vi "pp_loadStimParam.vi"(0 "error in (no error)":errorcluster) -> (5 "error out":errorcluster, 8 "Path":path, 14 "Total Trials":i32, 15 "Trial Randomization":enum32{"50% exactly", "Radio Selection 2"}(radio), 18 "Stims 1":dbl[][](array[numeric]), 19 "Stims 2":dbl[][](array[numeric]))   [LabVIEW 2013]
uses:
  <vilib>/Utility/xml.llb/Read From XML File(array).vi
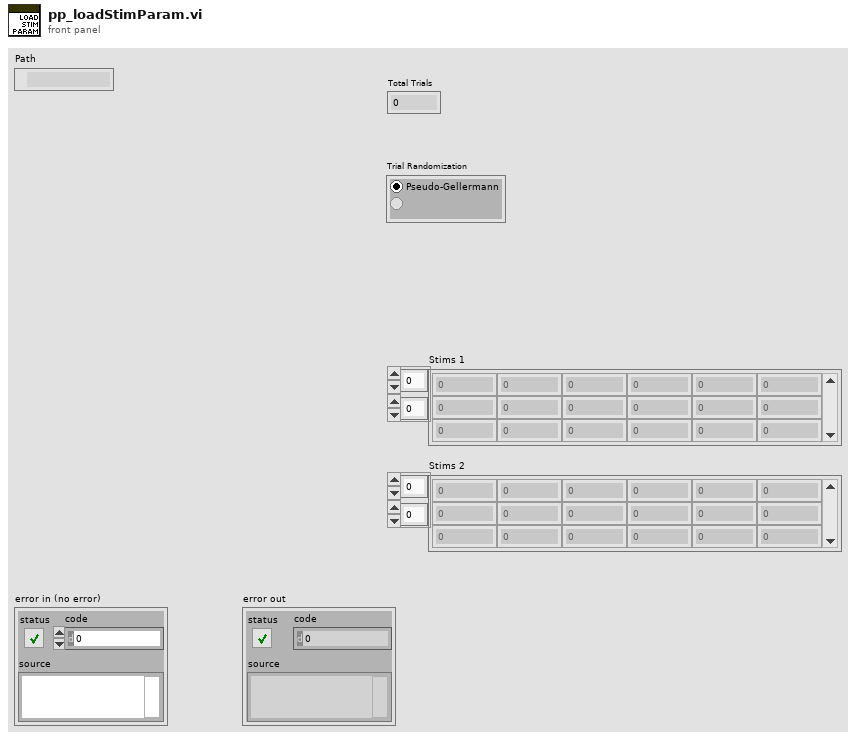
[diagram p1: front panel]
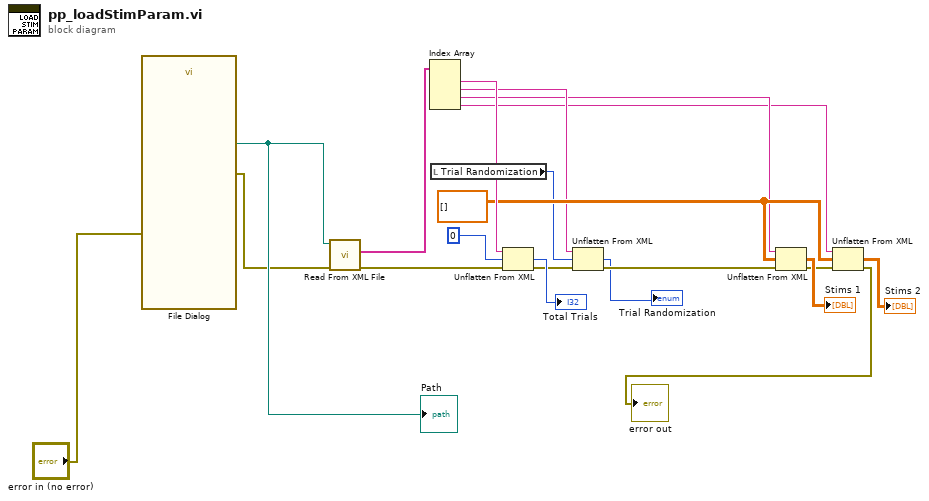
[diagram p0: block diagram]
diagram:
  w11 = dbl[][] [] ("Stims 1")
  n1 = call "File Dialog"("error in"="error in (no error)") -> ("selected path"=w19:path, "error out"=w18:errorcluster)  [unwired: 11 in, 2 out]
  "Path" <- w19
  n2 = call-poly <vilib>:"Read From XML File.vi"("error in (no error)"=w18, "XML File Path"=w19) -> ("error out"=w16:errorcluster, "XML Elements"=w20:string[])  [unwired: 7 in, 1 out]
  n3 = Index Array(array=w20) -> (element #1=w15:string, element #2=w10:string, element #3=w3:string, element #4=w2:string)  [unwired: 4 in]
  n4 = local read "Trial Randomization"() -> (w5:enum32{"50% exactly", "Radio Selection 2"})
  n5 = Unflatten From XML(xml string=w15, type=0, error in (no error)=w16) -> (value=→"Total Trials":i32, error out=w8:errorcluster)
  n6 = Unflatten From XML(xml string=w10, type=w5, error in (no error)=w8) -> (value=→"Trial Randomization":enum32{"50% exactly", "Radio Selection 2"}, error out=w4:errorcluster)
  n7 = Unflatten From XML(xml string=w3, type=w11, error in (no error)=w4) -> (value=→"Stims 1":dbl[][], error out=w7:errorcluster)
  n8 = Unflatten From XML(xml string=w2, type=w11, error in (no error)=w7) -> (value=→"Stims 2":dbl[][], error out=→"error out":errorcluster)
